vi "Compute Decay & Time Gates Wrapper.vi"(8 "error in (no error)":errorcluster, 11 "VI in":refnum<vi>) -> (0 "error out":errorcluster, 1 "Decay & Gates Plot String":string, 2 "Added Plot Name(s)":string, 3 "Decay Analysis Results":T2 {"A" format="%#_5g"; "tau" format="%#_4e"; "Bkgd" format="%#_4e"; "Min" format="%#_4e"; "Max" format="%#_4e"})   [LabVIEW 2019]
uses:
  Gate Analysis Results.ctl
  Decay & Gates Options.ctl
  <vilib>/Utility/High Resolution Relative Seconds.vi
panel:
  in  "Decay & Gates Options":T1
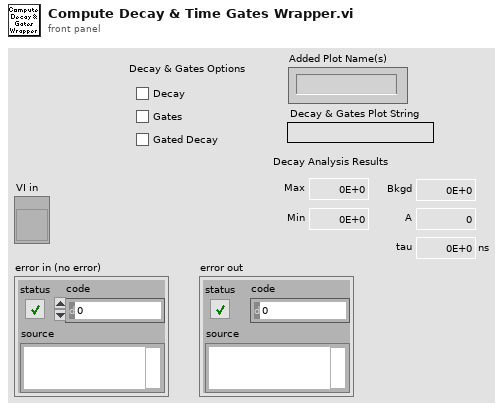
[diagram p1: front panel]
types:
  T1 = typedef "Decay & Gates Options.ctl" = cluster{"Decay":bool, "Gate":bool, "Gated Decay":bool}
  T2 = typedef "Gate Analysis Results.ctl" = cluster{"Max":dbl, "Min":dbl, "Bkgd":dbl, "tau ":dbl[unit], "A":dbl}
  T3 = typedef "SEPL Parameters.ctl" = cluster{"Display Parameters":T4, "Phasor Parameters":T6, "Decay & IRF Parameters":T9, "Gate Parameters":T11, "Detector Parameters":T13}
  T4 = typedef "Phasor Explorer Display Parameters.ctl" = cluster{"# Points":i32, "Ramp Type":enum16{"Linear", "Logarithmic"}, "Type of Series":T5, "Min tau":dbl[unit], "Max tau":dbl[unit], "Include 0":bool, "Include Infinity":bool}
  T5 = typedef "Type of Series.ctl" = enum16{"1-Exp Decays", "Linear Combination of 1-Exp"}
  T6 = typedef "Phasor Explorer Phasor Parameters.ctl" = cluster{"Harmonic frequency":dbl[unit], "Use f* = 1/D Frequency":bool, "Calibrated Phasor":bool, "Calibration Lifetime":dbl[unit], "Phasor Calculation":T7, "SEPL Type":T8, "# Gates":dbl, "Square Gate Width":dbl[unit], "Show Ticks":bool}
  T7 = typedef "Phasor Calculation Type.ctl" = enum16{"Direct Sum", "Analytical Formula"}
  T8 = typedef "SEPL Type.ctl" = enum16{"UC", "L_N", "L_N[W]"}
  T9 = typedef "Phasor Explorer Decay Parameters.ctl" = cluster{"Lifetime":dbl[unit], "IRF Offset":dbl[unit], "IRF Period":dbl[unit], "Normalized Decays":bool, "IRF Model":T10, "IRF Parameter 1":dbl[unit]}
  T10 = typedef "IRF Model.ctl" = enum16{"Dirac", "Exponential"}
  T11 = typedef "Phasor Explorer Gate Parameters.ctl" = cluster{"First Gate Start":dbl[unit], "Use Gate Center":bool, "Gate Width":dbl[unit], "Gate Step":dbl[unit], "# Gates":dbl, "Gate Type":T12, "Edge Width":dbl[unit], "Top Slope":dbl[unit], "Reversed Sawtooth?":bool, "Analytical Computation":bool, "Integration":enum32{"Item 0", "Item 1"}, "Tolerance":dbl, "# Steps":dbl, "Type of User-defined Function":enum32{"Gate", "IRF"}, "Use Gate Step":bool}
  T12 = typedef "Gate Type.ctl" = enum16{"Square", "Finite Edge Square", "Finite Edge, Tilted Top Square", "Triangle", "Sawtooth", "User-defined"}
  T13 = typedef "Phasor Explorer Detector Parameters.ctl" = cluster{"Frames/Image":i32, "Gates/Frame":i32, "Bits/Frame":i32, "Multiplicity":i32, "Incident Signal":dbl, "Poisson Signal":bool}
  T14 = typedef "Gate Definitions.ctl" = cluster{"First Gate: t1":ext, "Gate Width: W":ext, "Gate Step: d":ext, "# Gates: G":ext, "Use Gate Center":bool, "Frames/Image: F":i32, "Gates/Frame: L":i32, "Bits/Frame: q":i32, "Multiplicity: p":i32, "Gate Type":T12, "Gate Edge s":ext, "Gate Top Slope":ext, "Reversed Sawtooth?":bool, "Computation":bool, "User-defined Gate":T15, "Tolerance":ext, "Integration":enum32{"Item 0", "Item 1"}, "# Steps":ext, "Type of User-defined Function":enum32{"Gate", "IRF"}}
  T15 = typedef "XY Plot Data.ctl" = cluster{"X Array":dbl[], "Y Array":dbl[]}
  T16 = typedef "Decay Definiton.ctl" = cluster{"offset: t0":ext, "period: T":ext, "lifetime: tau":ext, "Incident Signal: I":ext, "Normalized Decays":bool, "IRF Model":T10, "IRF Parameter 1":ext, "Poisson Signal":bool}
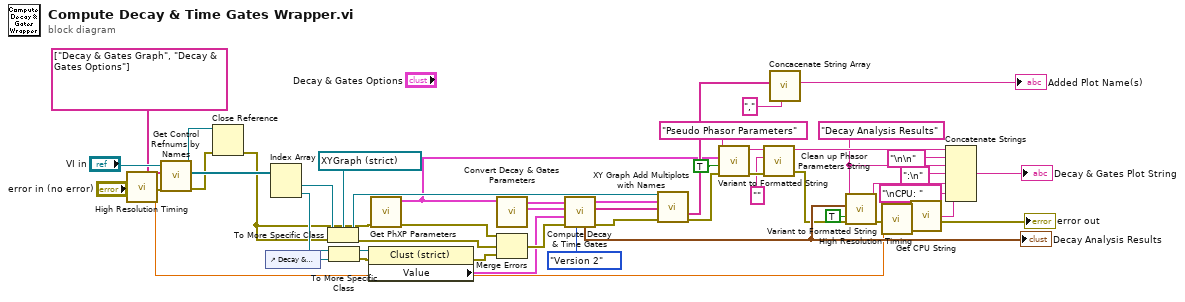
[diagram p0: block diagram]
diagram:
  w16 = "Decay Analysis Results" ("Label")
  n1 = call "High Resolution Timing.vi"("Error In"="error in (no error)") -> ("elapsed (relative) seconds"=w6:dbl, "Error Out"=w8:errorcluster)  [unwired: 16 in, 1 out]
  n2 = call "Get Control Refnums by Names.vi"("error in"=w8, "Control Labels"=string[] ["Decay & Gates Graph", "Decay & Gates Options"], "VI  Ref"="VI in") -> ("error out"=w2:errorcluster, "Ctl Refnums"=w51:refnum<vi>[], "VI  Ref (out)"=w46:refnum<vi>)  [unwired: 5 in, 1 out]
  n3 = Close Reference(reference=w46, error in (no error)=w2) -> (error out=w1:errorcluster)
  n4 = control-ref of="Decay & Gates Options"() -> (w38:refnum<vi>)
  n5 = Index Array(array=w51) -> (element #1=w50:refnum<vi>, element #2=w13:refnum<vi>)  [unwired: 2 in]
  n6 = To More Specific Class(target class=refnum<vi> refnum ("XYGraph in"), reference=w50, error in=w1) -> (specific class reference=w43:refnum<vi>, error out=w45:errorcluster)
  n7 = To More Specific Class(target class=w38, reference=w13) -> (specific class reference=w37:refnum<vi>, error out=w36:errorcluster)  [unwired: 1 in]
  n8 = property class="Clust (strict)"(reference=w37, error in=w36) -> (error out=w34:errorcluster, "Value"=w35:T1)  [unwired: 1 out]
  n9 = call "Get PhXP Parameters.vi"("Error In"=w1) -> ("Error Out"=w12:errorcluster, "Phasor Explorer Parameters"=w14:T3)  [unwired: 7 in, 2 out]
  n10 = call "Convert Decay & Gates Parameters.vi"("Phasor Parameters"=w14) -> ("Gates Definitions"=w44:T14, "Decay Definition"=w42:T16)  [unwired: 9 in]
  n11 = Merge Errors(w12, w45, w34) -> (w40:errorcluster)
  n12 = call "Compute Decay & Time Gates.vi"("Version"=enum32{"Version 1", "Version 2"}."Version 2", "Error In"=w40, "Decay & Gates Options"=w35, "Gates Definitions"=w44, "Decay Definition"=w42) -> ("Error Out"=w41:errorcluster, "Plot Names"=w10:string[], "Plots"=w11:cluster{"t Array":dbl[], "Gate Array":dbl[]}[], "Decay Analysis Results"=w27:T2)  [unwired: 3 out]
  "Decay Analysis Results" <- w27
  n13 = call "XY Graph Add Multiplots with Names.vi"("XYGraph in"=w43, "Array of Plots"=w11, "Array of Plot Names (\"Plot\")"=w10, "error in (no error)"=w41) -> ("Added Plot Names"=w21:string[], "error out"=w29:errorcluster)  [unwired: 7 in, 3 out]
  n14 = call "Variant to Formatted String.vi"("Error In"=w29, "Hide Long Cluster Names (T)"=TRUE ("Hide Long Names (Cluster)"), "Variant"=w14, "Label"="Pseudo Phasor Parameters") -> ("Error Out"=w30:errorcluster, "String"=w31:string)  [unwired: 6 in]
  n15 = call "Clean up Phasor Parameters String.vi"("Error In"=w30, "Cluster Label"="", "String in"=w31) -> ("Error Out"=w26:errorcluster, "String out"=w28:string)  [unwired: 7 in]
  n16 = call "Concacenate String Array.vi"("Separator (TAB)"=",", "String Array"=w21) -> ("Formatted String"=→"Added Plot Name(s)":string)  [unwired: 9 in]
  n17 = call "Variant to Formatted String.vi"("Error In"=w26, "Hide Long Cluster Names (T)"=TRUE ("Hide Long Names (Cluster)"), "Variant"=w27, "Label"=w16) -> ("Error Out"=w20:errorcluster, "String"=w24:string)  [unwired: 6 in]
  n18 = call "High Resolution Timing.vi"("relative seconds (NaN)"=w6, "Error In"=w20) -> ("elapsed (relative) seconds"=w5:dbl, "Error Out"=→"error out":errorcluster)  [unwired: 15 in, 1 out]
  n19 = call "Get CPU String.vi"("CPU (s)"=w5) -> ("String"=w3:string)  [unwired: 8 in]
  n20 = Concatenate Strings(w28, "\n\n" ("string"), w16, ":\n" ("string"), w24, "\nCPU: " ("string"), w3) -> (→"Decay & Gates Plot String":string)
